vi "Construct Field by Parsing Ctrl Label.vi"(8 "error in (no error)":errorcluster, 11 "Field in":refnum<class "Field.lvclass">) -> (0 "error out":errorcluster, 3 "Field out":refnum<class "Field.lvclass">)   [LabVIEW 2020, in "Old Field.lvlib" / "Field.lvclass"]
uses:
  Field.lvclass
  Field.lvclass/Field.ctl
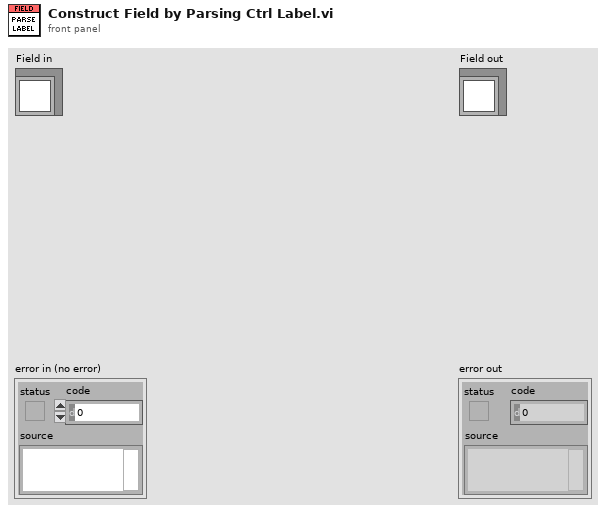
[diagram p1: front panel]
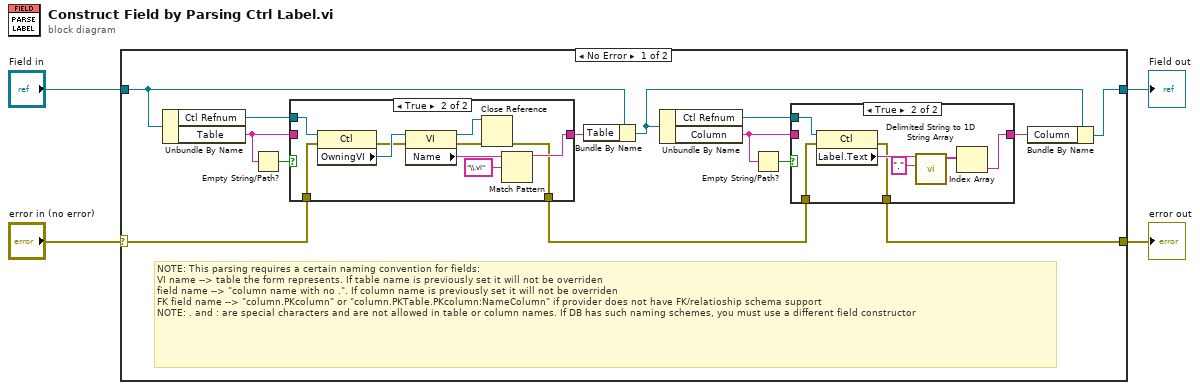
[diagram p0: block diagram]
diagram:
  n1 = case shown="No Error" "error in (no error)" {
    selector: "error in (no error)" -> [w15 w41]
    tunnel: [w5 w41] -> w3
    tunnel: [w7 w40] -> w1
    tunnel: "Field in" -> [w18 w40]
    frame No Error {
      # "NOTE: This parsing requires a certain naming convention for fields: \nVI name --> table the form represents. If table name is previously set it will not be overriden\nfield name --> \"column name with no .\". If column name is previously set it will not be overriden\nFK field name --> \"column.PKcolumn\" or \"column.PKTable.PKcolumn:NameColumn\" if provider does not have FK/relatioship schema support\nNOTE: . and : are special characters and are not allowed in table or column names. If DB has such naming schemes, you must use a different field constructor"
      n2 = Unbundle By Name(w18) -> ("Ctl Refnum"=w16:refnum<vi>, "Table"=w14:string)
      n3 = Empty String/Path?(string/path=w14) -> (empty?=w17:bool)
      n4 = case shown="True" w17 {
        tunnel: w16 -> [_ w33]
        tunnel: w15 -> [w28 w32]
        tunnel: w14 -> [w29 _]
        tunnel: [w29 w31] -> w13
        tunnel: [w28 w30] -> w6
        frame False {
        }
        frame True {
          n5 = property class="Ctl"(reference=w33, error in=w32) -> (error out=w37:errorcluster, "OwningVI"=w39:refnum<vi>)  [unwired: 1 out]
          n6 = property class="VI"(reference=w39, error in=w37) -> (reference out=w38:refnum<vi>, error out=w36:errorcluster, "Name"=w35:string)
          n7 = Close Reference(reference=w38, error in (no error)=w36) -> (error out=w30:errorcluster)
          n8 = Match Pattern(string=w35, regular expression="\\.vi") -> (before substring=w31:string)  [unwired: 1 in, 3 out]
        }
      }
      n9 = Bundle By Name(cluster=w18, "Table"=w13) -> (w9:refnum<class "Field.lvclass">)
      n10 = Unbundle By Name(w9) -> ("Ctl Refnum"=w11:refnum<vi>, "Column"=w10:string)
      n11 = Empty String/Path?(string/path=w10) -> (empty?=w12:bool)
      n12 = case shown="True" w12 {
        tunnel: w11 -> [_ w27]
        tunnel: w10 -> [w20 _]
        tunnel: [w20 w23] -> w8
        tunnel: w6 -> [w19 w22]
        tunnel: [w19 w21] -> w5
        frame False {
        }
        frame True {
          n13 = property class="Ctl"(reference=w27, error in=w22) -> (error out=w21:errorcluster, "Label.Text"=w25:string)  [unwired: 1 out]
          n14 = call <vilib>:"Delimited String to 1D String Array.vi"("delimiter"=".", "delimited string"=w25) -> ("string array"=w24:string[])  [unwired: 9 in]
          n15 = Index Array(array=w24) -> (element=w23:string)  [unwired: 1 in]
        }
      }
      n16 = Bundle By Name(cluster=w9, "Column"=w8) -> (w7:refnum<class "Field.lvclass">)
    }
    frame Error {
    }
  }
  "error out" <- w3
  "Field out" <- w1
